vi "Password_String.vi"(11 "Password":string) -> (3 "String":string)   [LabVIEW 2018]
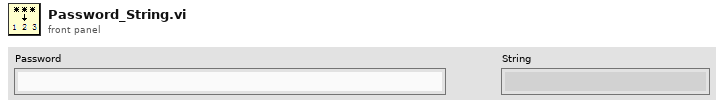
[diagram p1: front panel]
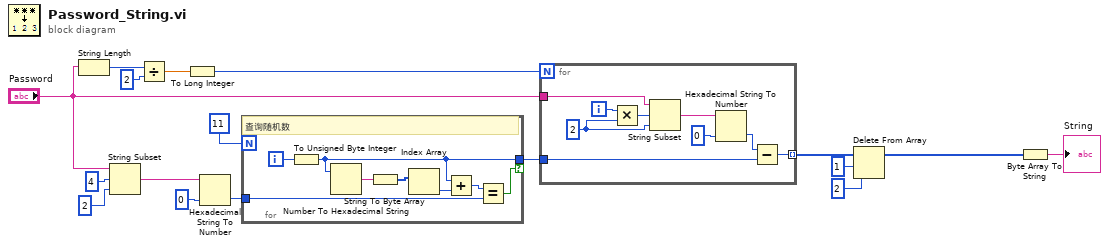
[diagram p0: block diagram]
diagram:
  n1 = String Length(string="Password") -> (length=w17:i32)
  n2 = String Subset(string="Password", offset (0)=4 ("偏移量(0)"), length (rest)=2 ("长度（剩余）")) -> (substring=w10:string)
  n3 = Divide(x=w17, y=2) -> (x/y=w15:dbl)
  n4 = To Long Integer(number=w15) -> (32bit integer=w7:i32)
  n5 = Hexadecimal String To Number(string=w10, default (0uL)=u8 0 ("默认(0 U32)")) -> (number=w9:u8)  [unwired: 1 in, 1 out]
  n6 = for {
    N: 11 -> [_]
    tunnel: w9 -> [w19]
    tunnel: [w21] -> w6 if=w18
    i -> [w23]
    # "查询随机数"
    n7 = To Unsigned Byte Integer(number=w23) -> (unsigned 8bit integer=w21:u8)
    n8 = Number To Hexadecimal String(2:w21) -> (0:w25:string)  [unwired: 1 in]
    n9 = String To Byte Array(string=w25) -> (unsigned byte array=w24:u8[])
    n10 = Index Array(array=w24) -> (element=w22:u8)  [unwired: 1 in]
    n11 = Add(x=w21, y=w22) -> (x+y=w20:u8)
    n12 = Equal?(x=w20, y=w19) -> (x = y?=w18:bool)
  }
  n13 = for {
    N: w7 -> [_]
    tunnel: "Password" -> [w34]
    tunnel: [w26] -> w5 mode=indexing
    tunnel: w6 -> [w27]
    i -> [w33]
    w31 = 2 ("y")
    n14 = Multiply(x=w33, y=w31) -> (x*y=w32:i32)
    n15 = String Subset(string=w34, offset (0)=w32, length (rest)=w31) -> (substring=w30:string)
    n16 = Hexadecimal String To Number(string=w30, default (0uL)=u8 0 ("默认(0 U32)")) -> (number=w28:u8)  [unwired: 1 in, 1 out]
    n17 = Subtract(x=w28, y=w27) -> (x-y=w26:u8)
  }
  n18 = Delete From Array(array=w5, length=1 ("长度"), index=2 ("索引")) -> (array with subset deleted=w1:u8[])  [unwired: 1 out]
  n19 = Byte Array To String(unsigned byte array=w1) -> (string=→"String":string)
